vi "获取vi引用.vi"(8 "error in":errorcluster, 11 "urlStr":string) -> (0 "error out":errorcluster, 2 "viPath":path, 3 "VIOut":refnum<vi>)   [LabVIEW 2014]
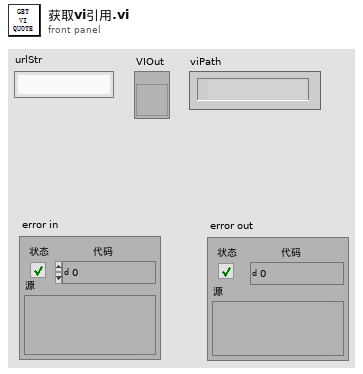
[diagram p1: front panel]
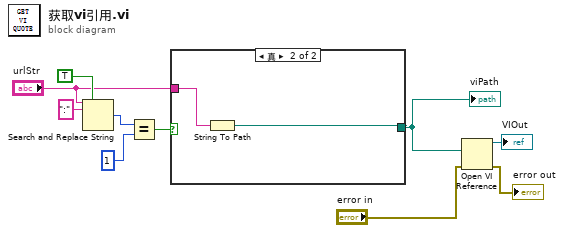
[diagram p0: block diagram]
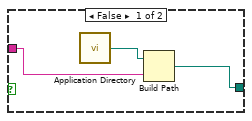
[diagram p2: hidden frame]
diagram:
  n1 = Search and Replace String(replace all?=TRUE ("替换全部？(F)"), input string="urlStr", search string=":" ("搜索字符串")) -> (number of replacements=w8:i32)  [unwired: 5 in, 3 out]
  n2 = Equal?(x=w8, y=1) -> (x = y?=w6:bool)
  n3 = case shown="真" w6 {
    tunnel: "urlStr" -> [w12 w15]
    tunnel: [w11 w14] -> w4
    frame False {
      n4 = call <vilib>:"Application Directory.vi"() -> ("Application Directory"=w13:path)
      n5 = Build Path(base path=w13, name or relative path=w12) -> (appended path=w11:path)
    }
    frame True {
      n6 = String To Path(string=w15) -> (path=w14:path)
    }
  }
  "viPath" <- w4
  n7 = Open VI Reference(vi path=w4, error in (no error)="error in") -> (vi reference=→"VIOut":refnum<vi>, error out=→"error out":errorcluster)  [unwired: 4 in]
